vi "Train Tip SVM.vi"(5 "Model Options":T1={"SVM Model"=enum."C-SVC", "Tolerance"=0.001, "Max. Iteration"=100000, "Nu"=0.1, "Shrinking"=TRUE, "Cost"=1.0, "Weighted Cost"=[]}, 7 "Kernel Options":T2={"Kernel"=enum."RBF", "Degree"=3, "Gamma"=1.0, "Coefficient"=0.0, "Sigma"=1.0, "Cache(MB)"=10.0}, 8 "error in (no error)":errorcluster, 9 "Classifier File":path=path "C:/Users/Andrew/Documents/Apatite to Zircon Code/Track Finding/TipClassifier.svm", 10 "Non-tip Data File":path=path "C:/Users/Andrew/Documents/Apatite to Zircon Code/Track Finding/Non-tip Data.csv", 11 "Tip Data File":path=path "C:/Users/Andrew/Documents/Apatite to Zircon Code/Track Finding/Tip Data.csv") -> (0 "error out":errorcluster, 2 "Non-tip Classification Accuracy":dbl, 3 "Tip Classification Accuracy":dbl)   [LabVIEW 2013]
uses:
  <vilib>/vision/Classification.llb/IMAQ SVM Kernel Options.ctl
  <vilib>/vision/Classification.llb/IMAQ SVM Model Options.ctl
  <vilib>/Utility/file.llb/Read From Spreadsheet File (DBL).vi
  <vilib>/vision/NI_Vision_Development_Module.lvlib
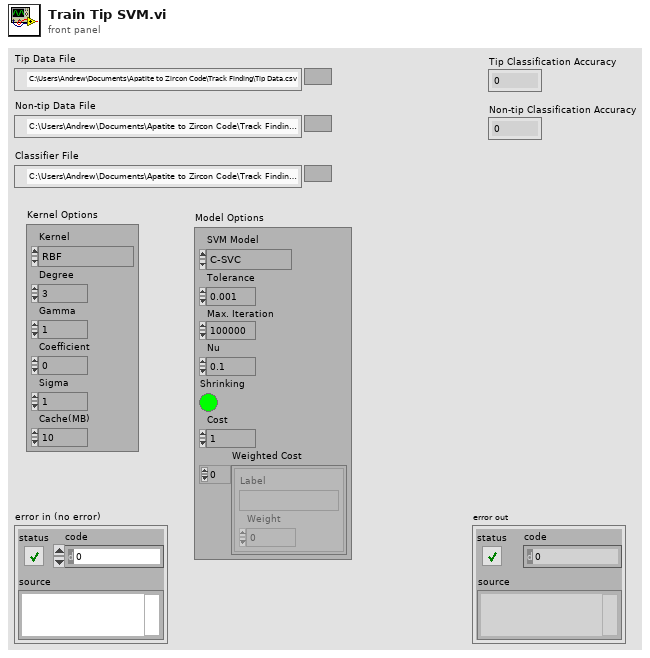
[diagram p1: front panel]
types:
  T1 = typedef "IMAQ SVM Model Options.ctl" = cluster{"SVM Model":enum32{"C-SVC", "nu-SVC", "One Class"}, "Tolerance":dbl, "Max. Iteration":i32, "Nu":dbl, "Shrinking":bool, "Cost":dbl, "Weighted Cost":cluster{"Label":string, "Weight":dbl}[]}
  T2 = typedef "IMAQ SVM Kernel Options.ctl" = cluster{"Kernel":enum32{"Linear", "Polynomial", "Gaussian", "RBF"}, "Degree":i32, "Gamma":dbl, "Coefficient":dbl, "Sigma":dbl, "Cache(MB)":dbl}
  T3 = typedef "Image Type" = u32
  T4 = typedef "IMAQ Image.ctl" = refnum<image>
  T5 = typedef "IMAQ Classifier Session.ctl" = refnum<k1>
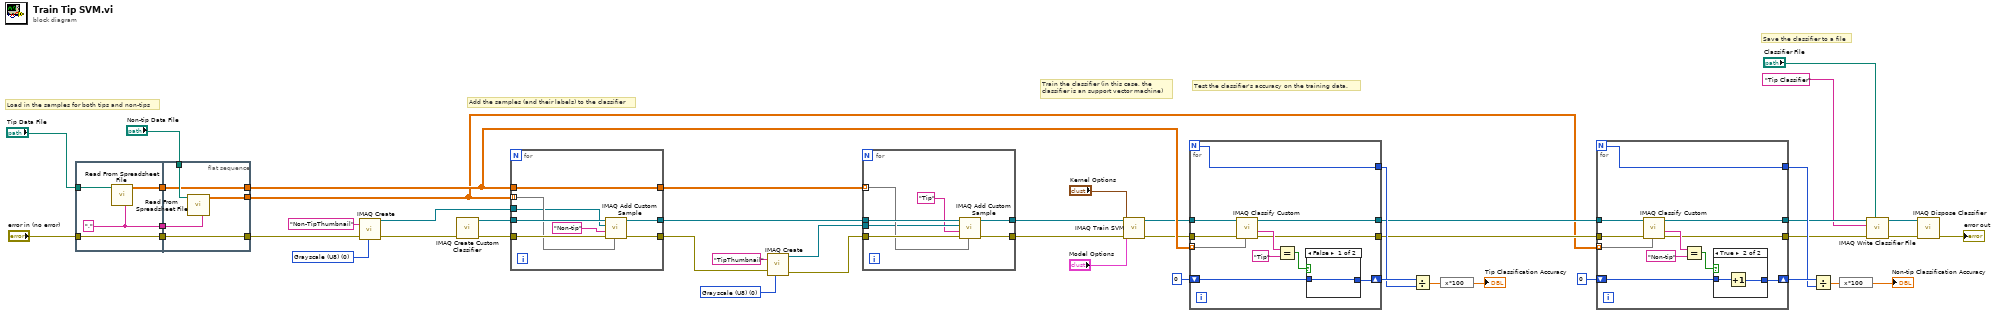
[diagram p0: block diagram]
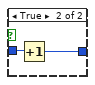
[diagram p3: hidden frame]
diagram:
  w36 = T3 0 items=["Grayscale (U8)", "Grayscale (I16)", "Grayscale (SGL)", "Complex (CSG)", "RGB (U32)", "HSL (U32)", "RGB (U64)", "Grayscale (U16)"] ("Image Type")
  w38 = T3 0 items=["Grayscale (U8)", "Grayscale (I16)", "Grayscale (SGL)", "Complex (CSG)", "RGB (U32)", "HSL (U32)", "RGB (U64)", "Grayscale (U16)"] ("Image Type")
  # "Save the classifier to a file"
  # "Test the classifier's accuracy on the training data."
  # "Train the classifier (in this case, the \nclassifier is an support vector machine)"
  # "Add the samples (and their labels) to the classifier"
  # "Load in the samples for both tips and non-tips"
  n1 = flat-sequence {
    tunnel: "Tip Data File" -> [w51]
    tunnel: "error in (no error)" -> [w50]
    tunnel: [w50] -> w45
    tunnel: [w49] -> w43
    tunnel: [w48] -> w31
    tunnel: [w56] -> w34
    tunnel: w45 -> [w56]
    tunnel: "Non-tip Data File" -> [w55]
    tunnel: [w54] -> w24
    tunnel: w43 -> [w53]
    tunnel: [w53] -> w30
    tunnel: w31 -> [w52]
    frame #0 {
      w48 = "," ("delimiter (\\t)")
      n2 = call-poly <vilib>:"Read From Spreadsheet File.vi"("delimiter (\\t)"=w48, "file path (dialog if empty)"=w51) -> ("all rows"=w49:dbl[][])  [unwired: 5 in, 4 out]
    }
    frame #1 {
      n3 = call-poly <vilib>:"Read From Spreadsheet File.vi"("delimiter (\\t)"=w52, "file path (dialog if empty)"=w55) -> ("all rows"=w54:dbl[][])  [unwired: 5 in, 4 out]
    }
  }
  n4 = call "IMAQ Create"("Image Name"="Non-TipThumbnail", "Image Type"=w36, "error in (no error)"=w34) -> ("New Image"=w14:T4, "error out"=w13:errorcluster)  [unwired: 2 in]
  n5 = call "IMAQ Create Custom Classifier"("error in (no error)"=w13) -> ("error out"=w41:errorcluster, "Classifier Session"=w42:T5)  [unwired: 9 in]
  n6 = for {
    tunnel: w24 -> [w62] mode=indexing
    tunnel: w42 -> [w63]
    tunnel: w41 -> [w64]
    tunnel: [w61] -> w39
    tunnel: [w60] -> w33
    tunnel: w30 -> [w59]
    tunnel: [w59] -> w40
    tunnel: w14 -> [w57]
    n7 = call "IMAQ Add Custom Sample"("Feature Vector"=w62, "error in (no error)"=w64, "Class"="Non-tip", "Image"=w57, "Classifier Session"=w63) -> ("error out"=w60:errorcluster, "Classifier Session (dup)"=w61:T5)  [unwired: 5 in]
  }
  n8 = call "IMAQ Create"("Image Name"="TipThumbnail", "Image Type"=w38, "error in (no error)"=w33) -> ("New Image"=w12:T4, "error out"=w11:errorcluster)  [unwired: 2 in]
  n9 = for {
    tunnel: w40 -> [w69] mode=indexing
    tunnel: w39 -> [w70]
    tunnel: w11 -> [w71]
    tunnel: [w68] -> w19
    tunnel: [w67] -> w18
    tunnel: w12 -> [w66]
    n10 = call "IMAQ Add Custom Sample"("Feature Vector"=w69, "error in (no error)"=w71, "Class"="Tip", "Image"=w66, "Classifier Session"=w70) -> ("error out"=w67:errorcluster, "Classifier Session (dup)"=w68:T5)  [unwired: 5 in]
  }
  n11 = call "IMAQ Train SVM"("error in (no error)"=w18, "Model Options"="Model Options", "Kernel Options"="Kernel Options", "Classifier Session"=w19) -> ("error out"=w17:errorcluster, "Classifier Session (dup)"=w20:T5)  [unwired: 4 in, 2 out]
  n12 = for {
    N -> [w72]
    tunnel: w20 -> [w82]
    tunnel: w17 -> [w81]
    tunnel: w30 -> [w80] mode=indexing
    shift-right: [w75] -> w28
    shift-left: 0 -> [w76]
    tunnel: [w74] -> w25
    tunnel: [w73] -> w26
    tunnel: [w72] -> w27
    n13 = call "IMAQ Classify Custom"("Feature Vector"=w80, "error in (no error)"=w81, "Classifier Session"=w82) -> ("error out"=w74:errorcluster, "Class"=w79:string, "Classifier Session (dup)"=w73:T5)  [unwired: 3 in, 3 out]
    n14 = Equal?(x=w79, y="Tip") -> (x = y?=w77:bool)
    n15 = case shown="False" w77 {
      tunnel: w76 -> [w83 w85]
      tunnel: [w83 w84] -> w75
      frame False {
      }
      frame True {
        n16 = Increment(x=w85) -> (x+1=w84:i32)
      }
    }
  }
  n17 = Divide(x=w28, y=w27) -> (x/y=w10:dbl)
  n18 = expression code="x*100"(w10) -> (→"Tip Classification Accuracy":dbl)
  n19 = for {
    N -> [w86]
    tunnel: w26 -> [w96]
    tunnel: w25 -> [w95]
    tunnel: w24 -> [w94] mode=indexing
    shift-right: [w89] -> w22
    shift-left: 0 -> [w90]
    tunnel: [w88] -> w5
    tunnel: [w87] -> w6
    tunnel: [w86] -> w21
    n20 = call "IMAQ Classify Custom"("Feature Vector"=w94, "error in (no error)"=w95, "Classifier Session"=w96) -> ("error out"=w88:errorcluster, "Class"=w93:string, "Classifier Session (dup)"=w87:T5)  [unwired: 3 in, 3 out]
    n21 = Equal?(x=w93, y="Non-tip") -> (x = y?=w91:bool)
    n22 = case shown="True" w91 {
      tunnel: w90 -> [w97 w99]
      tunnel: [w97 w98] -> w89
      frame False {
      }
      frame True {
        n23 = Increment(x=w99) -> (x+1=w98:i32)
      }
    }
  }
  n24 = Divide(x=w22, y=w21) -> (x/y=w8:dbl)
  n25 = expression code="x*100"(w8) -> (→"Non-tip Classification Accuracy":dbl)
  n26 = call "IMAQ Write Classifier File"("File Path"="Classifier File", "error in (no error)"=w5, "Description"="Tip Classifier", "Classifier Session"=w6) -> ("error out"=w4:errorcluster, "Classifier Session (dup)"=w3:T5)  [unwired: 6 in]
  n27 = call "IMAQ Dispose Classifier"("error in (no error)"=w4, "Classifier Session"=w3) -> ("error out"=→"error out":errorcluster)  [unwired: 9 in]
